vi "Show Trajectory.vi"(8 "error in (no error)":errorcluster, 10 "Show?":bool, 11 "Trajectory Drawer in":refnum<class "Trajectory Drawer.lvclass">) -> (0 "error out":errorcluster, 3 "Trajectory Drawer out":refnum<class "Trajectory Drawer.lvclass">)   [LabVIEW 2013, in "Trajectory Drawer.lvclass"]
uses:
  Trajectory Drawer.lvclass
  Trajectory Drawer.lvclass/Trajectory Drawer.ctl
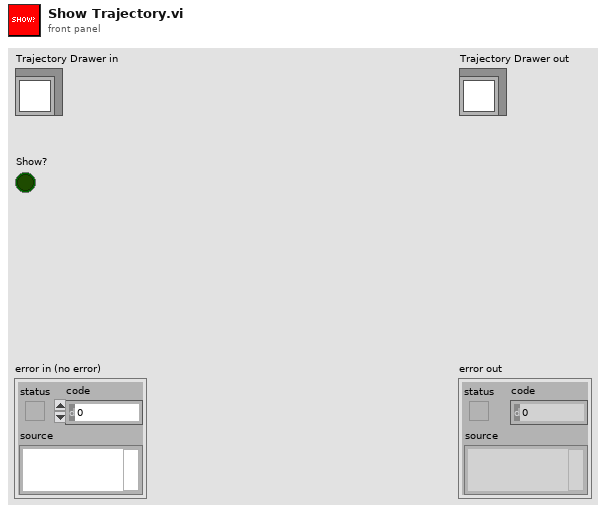
[diagram p1: front panel]
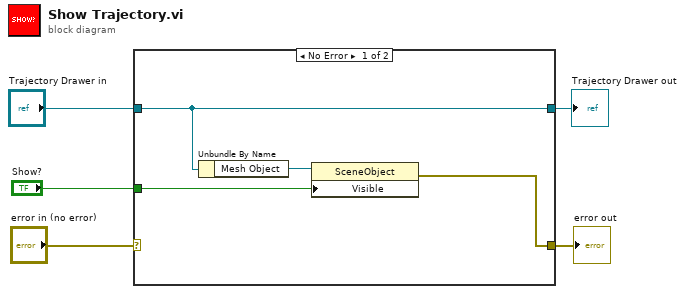
[diagram p0: block diagram]
diagram:
  n1 = case shown="No Error" "error in (no error)" {
    selector: "error in (no error)" -> [_ w11]
    tunnel: [w6 w11] -> w4
    tunnel: [w9 w10] -> w2
    tunnel: "Trajectory Drawer in" -> [w9 w10]
    tunnel: "Show?" -> [w7 _]
    frame No Error {
      n2 = Unbundle By Name(w9) -> ("Mesh Object"=w8:refnum<vi>)
      n3 = property class="SceneObject"(reference=w8, "Visible"=w7) -> (error out=w6:errorcluster)  [unwired: 1 in, 1 out]
    }
    frame Error {
    }
  }
  "error out" <- w4
  "Trajectory Drawer out" <- w2
